vi "Do.vi"(8 "error in":errorcluster, 10 "Actor in":refnum<class "Actor.lvclass">, 11 "Change Individual Power Supply MSG":refnum<class "Change Individual Power Supply MSG.lvclass">) -> (0 "error out":errorcluster, 2 "Actor out":refnum<class "Actor.lvclass">)   [LabVIEW 2014, in "Controller.lvlib" / "Change Individual Power Supply MSG.lvclass"]
doc: "(<B>Filename</B>: Actor Framework.lvlib:Message.lvclass:Do.vi)\n\nDefines what a message does when it is received by an actor. Generally, a message instructs an actor to invoke one of its methods. By default, this method does nothing. A child class must override it to define behavior. Create a child class by using the Actor Framework Message Maker dialog box."
uses:
  Change Individual Power Supply MSG.lvclass
  <vilib>/ActorFramework/Actor/Actor.lvclass
  Change Individual Power Supply MSG.lvclass/Change Individual Power Supply MSG.ctl
  Controller.lvclass
  SuperActor/Ex Nested.lvclass/Ex Nested.ctl
  SuperActor/Read CVT Session.vi
  SuperActor/Read Log Session.vi
  <vilib>/DAQmx/write.llb/DAQmx Write (Digital 1D Bool NChan 1Samp 1Line).vi
  <userlib>/_Session Fwk/Session - Root.lvclass
  reusable/Session APIs/Session Log/System Log.lvclass
  reusable/Session APIs/CVT/CVT.lvclass
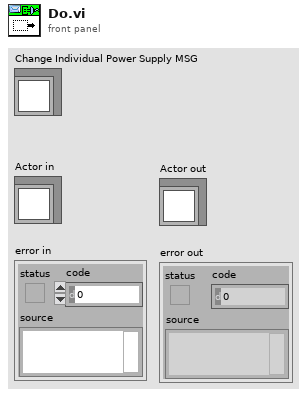
[diagram p1: front panel]
types:
  T1 = typedef "Session - Root.lvclass/Session Handle.ctl" = refnum<data-value>
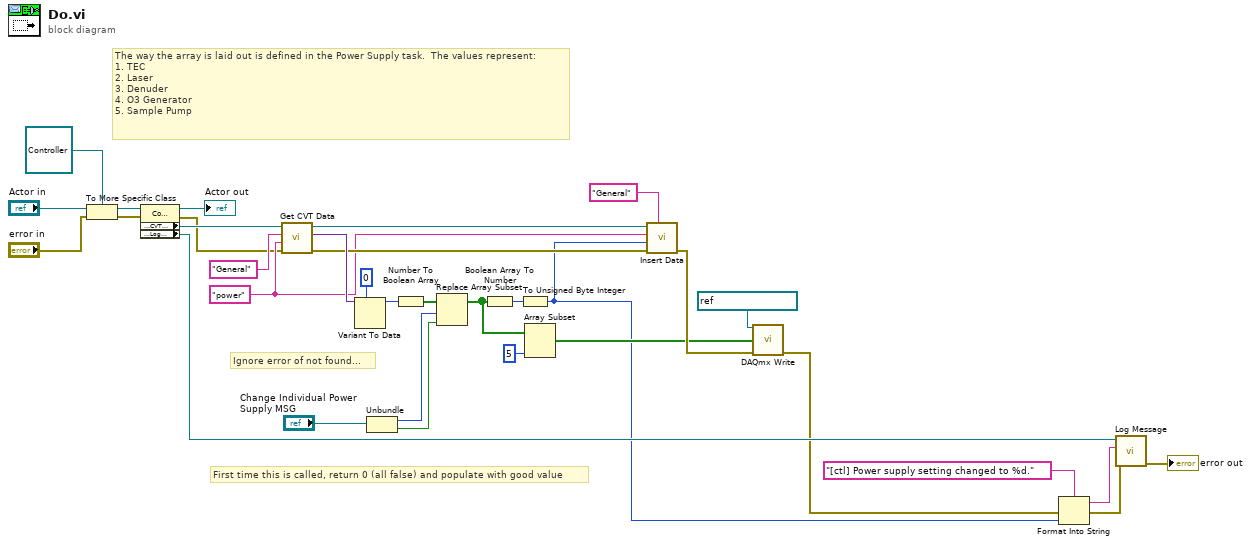
[diagram p0: block diagram]
diagram:
  w3 = "power" ("Group")
  # "First time this is called, return 0 (all false) and populate with good value"
  # "Ignore error of not found..."
  # "The way the array is laid out is defined in the Power Supply task.  The values represent:\n1. TEC\n2. Laser\n3. Denuder\n4. O3 Generator\n5. Sample Pump"
  n1 = To More Specific Class(target class=refnum<class "Controller.lvclass"> refnum ("Controller:Controller"), reference="Actor in", error in="error in") -> (specific class reference=w29:refnum<class "Controller.lvclass">, error out=w2:errorcluster)
  n2 = property class="Controller"(reference=w29, error in=w2) -> (reference out=→"Actor out":refnum<class "Controller.lvclass">, error out=w1:errorcluster, "Accessors:CVT Session"=w21:T1, "Accessors:Log Session"=w25:T1)
  n3 = call "Get CVT Data.vi"("error in"=w1, "Variable"=w3, "Group"="General", "CVT Session In"=w21) -> ("error out"=w11:errorcluster, "Data Out"=w18:variant, "CVT Session Out"=w20:T1)  [unwired: 4 in, 1 out]
  n4 = Variant To Data(type=u8 0, Variant=w18) -> (data=w16:u8)  [unwired: 1 in, 1 out]
  n5 = Unbundle("Change Individual Power Supply MSG") -> (w14:i32, w13:bool)
  n6 = Number To Boolean Array(number=w16) -> (Boolean array=w15:bool[])
  n7 = Replace Array Subset(array=w15, new element=w13, index=w14) -> (w9:bool[])
  n8 = Boolean Array To Number(Boolean array=w9) -> (number=w12:u32)
  n9 = To Unsigned Byte Integer(number=w12) -> (unsigned 8bit integer=w5:u8)
  n10 = Array Subset(array=w9, length=5) -> (w8:bool[])  [unwired: 1 in]
  n11 = call "Insert Data.vi"("Group"="General" ("tag"), "error in"=w11, "Data"=w5, "tag"=w3, "CVT Session In"=w20) -> ("error out"=w10:errorcluster)  [unwired: 5 in, 1 out]
  n12 = call-poly <vilib>:"DAQmx Write.vi"("task/channels in"=refnum<k21> "Power Supply", "data"=w8, "error in"=w10) -> ("error out"=w24:errorcluster)  [unwired: 10 in, 2 out]
  n13 = Format Into String(format string="[ctl] Power supply setting changed to %d.", error in=w24, w5) -> (resulting string=w27:string, error out=w23:errorcluster)  [unwired: 1 in]
  n14 = call "Log Message.vi"("error in"=w23, "MSG In"=w27, "session in"=w25) -> ("error out"=→"error out":errorcluster)  [unwired: 7 in, 1 out]
